vi "Send Visa Payload.vi"(8 "error in":errorcluster, 10 "Command":string, 11 "Local Resource in":refnum<visa-resource-name>) -> (0 "error out":errorcluster, 3 "Local Resource out":refnum<visa-resource-name>)   [LabVIEW 2019, in "6972A.lvlib" / "6972A.lvclass"]
uses:
  Library/6972A.lvclass
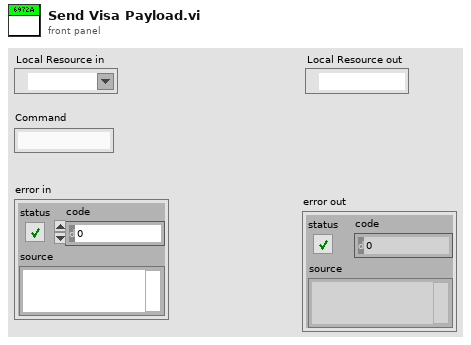
[diagram p1: front panel]
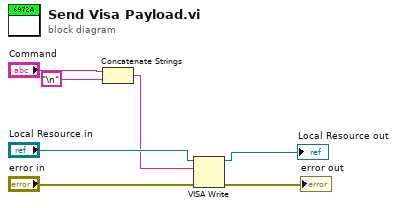
[diagram p0: block diagram]
diagram:
  n1 = Concatenate Strings("Command", "\n") -> (w3:string)
  n2 = VISA Write(VISA resource name="Local Resource in", write buffer=w3, error in (no error)="error in") -> (VISA resource name out=→"Local Resource out":refnum<visa-resource-name>, error out=→"error out":errorcluster)  [unwired: 1 out]
